vi "Method_Const.vi"(4 "Value":i64, 5 "Value A":refnum<class "Abs_I64 Integer.lvclass">) -> (1 "Result":refnum<class "Abs_Boolean.lvclass">)   [LabVIEW 2021, in "Less_I64.lvclass"]
uses:
  Less_I64.lvclass
  Abs_Types/I64 Integer/Abs_I64 Integer.lvclass
  C:/Program Files (x86)/National Instruments/LabVIEW 2021/vi.lib/TSA/Abstract Data Classes/Abs_Types/Numeric/Abs_Numeric.lvclass
  Abs_Types/Boolean/Abs_Boolean.lvclass
  C:/TSA/LV_Abstract/Source/Functions/Support/Compare/Two Term/I64/AbsComp_Two Term_I64.lvclass
  C:/Program Files (x86)/National Instruments/LabVIEW 2021/vi.lib/TSA/Abstract Data Classes/Abs_Types/Boolean/Abs_Boolean.lvclass
  Support/Compare/Two Term/I64/AbsComp_Two Term_I64.lvclass/AbsComp_Two Term_I64.ctl
  Support/Compare/Two Term/I64/Properties/Write Numeric A.vi
  Support/Compare/Two Term/I64/Properties/Write Numeric B.vi
  Constants/Support/I64/Const_I64.lvclass
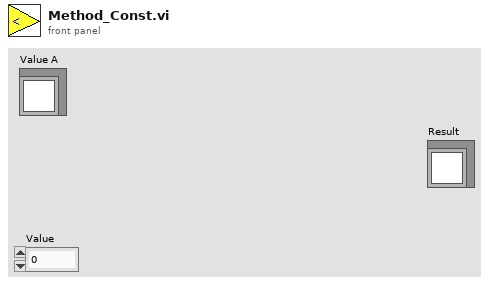
[diagram p1: front panel]
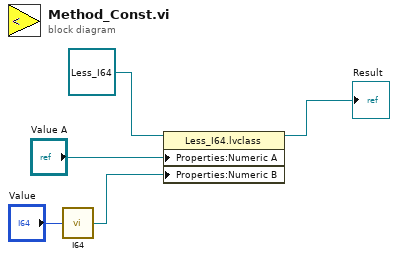
[diagram p0: block diagram]
diagram:
  n1 = call "I64.vi"("Value"="Value") -> ("Constant"=w2:refnum<class "Abs_I64 Integer.lvclass">)  [unwired: 4 in]
  n2 = property class="Less_I64.lvclass"(reference=refnum<class "Less_I64.lvclass"> refnum ("Greater 0_U64.lvclass"), "Properties:Numeric A"="Value A", "Properties:Numeric B"=w2) -> (reference out=→"Result":refnum<class "Less_I64.lvclass">)  [unwired: 1 in, 1 out]
